vi "Finish.vi"   [LabVIEW 2018]
doc: "This VI is called just before exiting. It is expected to close I/O refnum, save collected data, etc."
uses:
  <vilib>/Rock Robotics/WPI/Utilities/WPI_GetSetVariantRefNum.vi
types:
  T1 = typedef "WPI_JoystickDevRef.ctl" = cluster{"Device":T2}
  T2 = typedef "WPI_JoystickDeviceEnum.ctl" = enum16{"USB 0", "USB 1", "USB 2", "USB 3", "USB 4", "USB 5"}
  T3 = typedef "WPI_SolenoidDevRef.ctl" = cluster{"DevStatus":errorcluster, "Pneumatics Control Module":u8, "Forward Solenoid Channel":T4, "Reverse Solenoid Channel":T4}
  T4 = typedef "WPI_SolenoidChannel.ctl" = enum8{"Solenoid 0", "Solenoid 1", "Solenoid 2", "Solenoid 3", "Solenoid 4", "Solenoid 5", "Solenoid 6", "Solenoid 7", "Invalid"}
  T5 = typedef "WPI_MotorControlDeviceRef.ctl" = cluster{"DeviceStatus":errorcluster, "Type":T6, "PWM":cluster{"PWM Channel":T7, "DeadBand":T8}, "CAN":cluster{"Device Number":u8, "SetOutput VI Ref":variant, "GetOutput VI Ref":variant, "Enable VI Ref":variant, "Disable VI Ref":variant, "Data":variant}, "Invert":bool, "DIO PWM":cluster{"PWM \"Enable\" Channel":T7, "DIOChannel":T9, "PWM Rate":dbl}}
  T6 = typedef "WPI_MotorControlType.ctl" = enum16{"PWM", "CAN", "DIO PWM"}
  T7 = typedef "FPGA_DIOPWMChannel.ctl" = enum8{"PWM 0", "PWM 1", "PWM 2", "PWM 3", "PWM 4", "PWM 5", "PWM 6", "PWM 7", "PWM 8", "PWM 9", "PWM MXP 0", "PWM MXP 1", "PWM MXP 2", "PWM MXP 3", "PWM MXP 4", "PWM MXP 5", "PWM MXP 6", "PWM MXP 7", "PWM MXP 8", "PWM MXP 9", "Invalid"}
  T8 = typedef "WPI_PWMDeadband.ctl" = cluster{"Name":string, "maxPositivePwm":i32, "minPositivePwm":i32, "centerPwm":i32, "maxNegativePwm":i32, "minNegativePwm":i32, "angularRange":u16}
  T9 = typedef "FPGA_DIOChannel.ctl" = enum8{"DIO 0", "DIO 1", "DIO 2", "DIO 3", "DIO 4", "DIO 5", "DIO 6", "DIO 7", "DIO 8", "DIO 9", "DIO MXP 0", "DIO MXP 1", "DIO MXP 2", "DIO MXP 3", "DIO MXP 4", "DIO MXP 5", "DIO MXP 6", "DIO MXP 7", "DIO MXP 8", "DIO MXP 9", "DIO MXP 10", "DIO MXP 11", "DIO MXP 12", "DIO MXP 13", "DIO MXP 14", "DIO MXP 15", "SPI Port CS1", "SPI Port CS2", "SPI Port CS3", "SPI Port MISO", "SPI Port MOSI", "Invalid"}
  T10 = typedef "WPI_AnalogChannelDevRef.ctl" = cluster{"DevStatus":errorcluster, "Analog Channel":T11}
  T11 = typedef "FPGA_AIChannel.ctl" = enum8{"AI 0", "AI 1", "AI 2", "AI 3", "AI MXP 0", "AI MXP 1", "AI MXP 2", "AI MXP 3", "Invalid"}
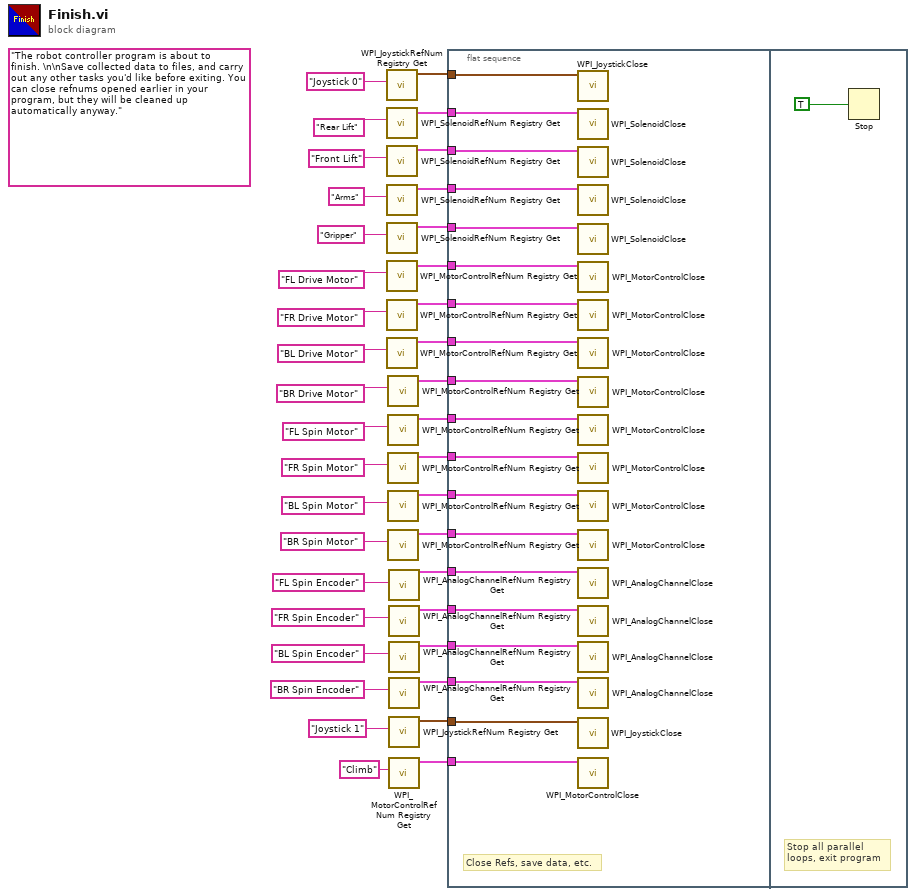
[diagram p0: block diagram]
diagram:
  (unwired) "The robot controller program is about to finish. \n\nSave collected data to files, and carry out any other tasks you'd like before exiting. You can close refnums opened earlier in your program, but they will be cleaned up automatically anyway."
  n1 = call <vilib>:"WPI_JoystickRefNum Registry Get.vi"("refnum name"="Joystick 0") -> ("JoystickDevRef"=w37:T1)  [unwired: 1 in, 9 out]
  n2 = call <vilib>:"WPI_SolenoidRefNum Registry Get.vi"("refnum name"="Rear Lift") -> ("SolenoidDevRef"=w32:T3)  [unwired: 9 in, 1 out]
  n3 = call <vilib>:"WPI_SolenoidRefNum Registry Get.vi"("refnum name"="Front Lift") -> ("SolenoidDevRef"=w31:T3)  [unwired: 9 in, 1 out]
  n4 = call <vilib>:"WPI_SolenoidRefNum Registry Get.vi"("refnum name"="Arms") -> ("SolenoidDevRef"=w30:T3)  [unwired: 9 in, 1 out]
  n5 = call <vilib>:"WPI_SolenoidRefNum Registry Get.vi"("refnum name"="Gripper") -> ("SolenoidDevRef"=w29:T3)  [unwired: 9 in, 1 out]
  n6 = call <vilib>:"WPI_MotorControlRefNum Registry Get.vi"("refnum name"="FL Drive Motor") -> ("MotorControlDevRef"=w19:T5)  [unwired: 9 in, 1 out]
  n7 = call <vilib>:"WPI_MotorControlRefNum Registry Get.vi"("refnum name"="FR Drive Motor") -> ("MotorControlDevRef"=w20:T5)  [unwired: 9 in, 1 out]
  n8 = call <vilib>:"WPI_MotorControlRefNum Registry Get.vi"("refnum name"="BL Drive Motor") -> ("MotorControlDevRef"=w18:T5)  [unwired: 9 in, 1 out]
  n9 = call <vilib>:"WPI_MotorControlRefNum Registry Get.vi"("refnum name"="BR Drive Motor") -> ("MotorControlDevRef"=w17:T5)  [unwired: 9 in, 1 out]
  n10 = call <vilib>:"WPI_MotorControlRefNum Registry Get.vi"("refnum name"="FL Spin Motor") -> ("MotorControlDevRef"=w16:T5)  [unwired: 9 in, 1 out]
  n11 = call <vilib>:"WPI_MotorControlRefNum Registry Get.vi"("refnum name"="FR Spin Motor") -> ("MotorControlDevRef"=w15:T5)  [unwired: 9 in, 1 out]
  n12 = call <vilib>:"WPI_MotorControlRefNum Registry Get.vi"("refnum name"="BL Spin Motor") -> ("MotorControlDevRef"=w14:T5)  [unwired: 9 in, 1 out]
  n13 = call <vilib>:"WPI_MotorControlRefNum Registry Get.vi"("refnum name"="BR Spin Motor") -> ("MotorControlDevRef"=w13:T5)  [unwired: 9 in, 1 out]
  n14 = call <vilib>:"WPI_AnalogChannelRefNum Registry Get.vi"("refnum name"="FL Spin Encoder") -> ("AIDeviceRef"=w8:T10)  [unwired: 9 in, 1 out]
  n15 = call <vilib>:"WPI_AnalogChannelRefNum Registry Get.vi"("refnum name"="FR Spin Encoder") -> ("AIDeviceRef"=w7:T10)  [unwired: 9 in, 1 out]
  n16 = call <vilib>:"WPI_AnalogChannelRefNum Registry Get.vi"("refnum name"="BL Spin Encoder") -> ("AIDeviceRef"=w6:T10)  [unwired: 9 in, 1 out]
  n17 = call <vilib>:"WPI_AnalogChannelRefNum Registry Get.vi"("refnum name"="BR Spin Encoder") -> ("AIDeviceRef"=w5:T10)  [unwired: 9 in, 1 out]
  n18 = call <vilib>:"WPI_JoystickRefNum Registry Get.vi"("refnum name"="Joystick 1") -> ("JoystickDevRef"=w4:T1)  [unwired: 1 in, 9 out]
  n19 = call <vilib>:"WPI_MotorControlRefNum Registry Get.vi"("refnum name"="Climb") -> ("MotorControlDevRef"=w2:T5)  [unwired: 9 in, 1 out]
  n20 = flat-sequence {
    tunnel: w37 -> [w57]
    tunnel: w32 -> [w56]
    tunnel: w31 -> [w55]
    tunnel: w30 -> [w54]
    tunnel: w29 -> [w53]
    tunnel: w20 -> [w52]
    tunnel: w19 -> [w51]
    tunnel: w18 -> [w50]
    tunnel: w17 -> [w49]
    tunnel: w16 -> [w48]
    tunnel: w15 -> [w47]
    tunnel: w14 -> [w46]
    tunnel: w13 -> [w45]
    tunnel: w8 -> [w44]
    tunnel: w7 -> [w43]
    tunnel: w6 -> [w42]
    tunnel: w5 -> [w41]
    tunnel: w4 -> [w40]
    tunnel: w2 -> [w39]
    frame #0 {
      # "Close Refs, save data, etc."
      n21 = call <vilib>:"WPI_JoystickClose.vi"("JoystickDevRef"=w57) -> ()  [unwired: 11 out]
      n22 = call <vilib>:"WPI_SolenoidClose.vi"("SolenoidDevRef"=w56) -> ()  [unwired: 10 in, 1 out]
      n23 = call <vilib>:"WPI_SolenoidClose.vi"("SolenoidDevRef"=w55) -> ()  [unwired: 10 in, 1 out]
      n24 = call <vilib>:"WPI_SolenoidClose.vi"("SolenoidDevRef"=w54) -> ()  [unwired: 10 in, 1 out]
      n25 = call <vilib>:"WPI_SolenoidClose.vi"("SolenoidDevRef"=w53) -> ()  [unwired: 10 in, 1 out]
      n26 = call <vilib>:"WPI_MotorControlClose.vi"("MotorControlDevRef"=w51) -> ()  [unwired: 10 in, 1 out]
      n27 = call <vilib>:"WPI_MotorControlClose.vi"("MotorControlDevRef"=w52) -> ()  [unwired: 10 in, 1 out]
      n28 = call <vilib>:"WPI_MotorControlClose.vi"("MotorControlDevRef"=w50) -> ()  [unwired: 10 in, 1 out]
      n29 = call <vilib>:"WPI_MotorControlClose.vi"("MotorControlDevRef"=w49) -> ()  [unwired: 10 in, 1 out]
      n30 = call <vilib>:"WPI_MotorControlClose.vi"("MotorControlDevRef"=w48) -> ()  [unwired: 10 in, 1 out]
      n31 = call <vilib>:"WPI_MotorControlClose.vi"("MotorControlDevRef"=w47) -> ()  [unwired: 10 in, 1 out]
      n32 = call <vilib>:"WPI_MotorControlClose.vi"("MotorControlDevRef"=w46) -> ()  [unwired: 10 in, 1 out]
      n33 = call <vilib>:"WPI_MotorControlClose.vi"("MotorControlDevRef"=w45) -> ()  [unwired: 10 in, 1 out]
      n34 = call <vilib>:"WPI_AnalogChannelClose.vi"("AIDeviceRef"=w44) -> ()  [unwired: 10 in, 1 out]
      n35 = call <vilib>:"WPI_AnalogChannelClose.vi"("AIDeviceRef"=w43) -> ()  [unwired: 10 in, 1 out]
      n36 = call <vilib>:"WPI_AnalogChannelClose.vi"("AIDeviceRef"=w42) -> ()  [unwired: 10 in, 1 out]
      n37 = call <vilib>:"WPI_AnalogChannelClose.vi"("AIDeviceRef"=w41) -> ()  [unwired: 10 in, 1 out]
      n38 = call <vilib>:"WPI_JoystickClose.vi"("JoystickDevRef"=w40) -> ()  [unwired: 11 out]
      n39 = call <vilib>:"WPI_MotorControlClose.vi"("MotorControlDevRef"=w39) -> ()  [unwired: 10 in, 1 out]
    }
    frame #1 {
      # "Stop all parallel\nloops, exit program"
      n40 = Stop(stop? (T)=TRUE ("Quit")) -> ()
    }
  }
